vi "GetPathByQualifiedName.vi"(8 "error in (no error)":errorcluster, 9 "Qualified name":string, 11 "CDependencyList in":refnum<class "CDependencyList.lvclass">) -> (0 "error out":errorcluster, 1 "Path":string, 2 "key found?":bool, 3 "CDependencyList out":refnum<class "CDependencyList.lvclass">)   [LabVIEW 2020, in "DependencyInspection.lvlib" / "CDependencyList.lvclass"]
uses:
  CDependencyList.lvclass
  CDependencyList.lvclass/CDependencyList.ctl
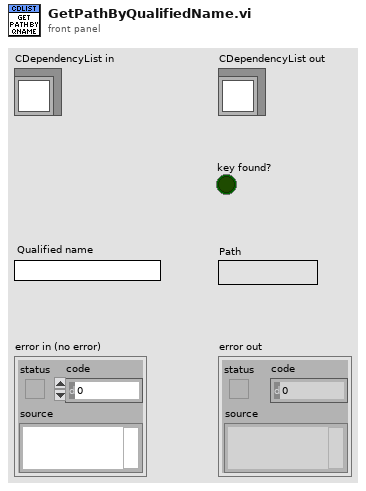
[diagram p1: front panel]
types:
  T1 = typedef "DependencyInspection.lvlib/CDependencyList.lvclass/QualifiedNamesToPathsMapRef.ctl" = refnum<data-value>
  T2 = typedef "DependencyInspection.lvlib/CDependencyList.lvclass/QualifiedNamesToPathsMap.ctl" = map{string, string}
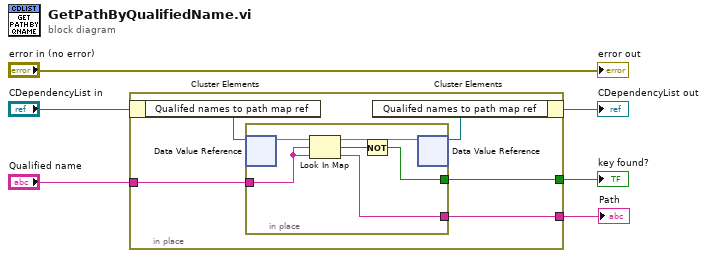
[diagram p0: block diagram]
diagram:
  n1 = in-place {
    in-place-border: "Qualified name" -> [w11]
    in-place-border: [w10] -> w4
    in-place-border: [w9] -> w1
    n2 = in-place-cluster #1("CDependencyList in") -> ("Qualifed names to path map ref"=w8:T1)
    n3 = in-place {
      in-place-border: w11 -> [w12]
      in-place-border: [w16] -> w10
      in-place-border: [w15] -> w9
      n4 = in-place-dvr #2(w8) -> (w13:T2)  [unwired: 1 out]
      n5 = Look In Map(map=w13, key=w12, default value=w12) -> (key not found?=w14:bool, value=w15:string)
      n6 = Not(x=w14) -> (.not. x?=w16:bool)
      n7 = in-place-dvr #2(w13) -> (w7:T1)  [unwired: 1 out]
    }
    n8 = in-place-cluster #1("Qualifed names to path map ref"=w7) -> (→"CDependencyList out":refnum<class "CDependencyList.lvclass">)
  }
  "key found?" <- w4
  "Path" <- w1
  "error out" <- "error in (no error)"
